vi "Stop.vi"(8 "error in (no error)":errorcluster) -> (0 "error out":errorcluster)   [LabVIEW 2017, in "VDMS_VibAPI.lvlib"]
uses:
  <vilib>/addons/InsightCM/Devices/Shared/Cms/Fpga/AcquisitionFpgaTach/source/subVIs/VibAPI/VDMS_VibAPI.lvlib
  <vilib>/rvi/eio/common/nirviEmuTemplateMethod_errors.vi
  <vilib>/eio/EIONode/EIONode.xnode
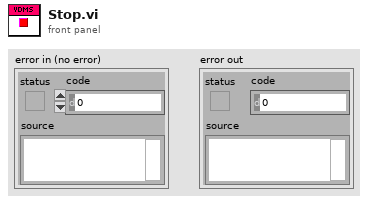
[diagram p1: front panel]
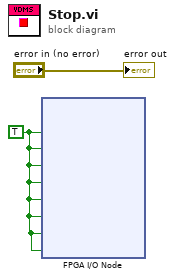
[diagram p0: block diagram]
diagram:
  w2 = TRUE ("Mod1/Stop")
  n1 = xnode "FPGA I/O Node"("Mod1/Stop"=w2, "Mod2/Stop"=w2, "Mod3/Stop"=w2, "Mod4/Stop"=w2, "Mod5/Stop"=w2, "Mod6/Stop"=w2, "Mod7/Stop"=w2, "Mod8/Stop"=w2) -> ()  [unwired: 9 in, 9 out]
  "error out" <- "error in (no error)"
